vi "Set initial rect size.vi"(8 "error in (no error)":errorcluster, 11 "Cam Session":T1) -> (0 "error out":errorcluster, 2 "Rectangle":T2, 3 "Session Out":T1)   [LabVIEW 2020]
uses:
  <vilib>/vision/driver/NI_Vision_Acquisition_Software.lvlib
  <vilib>/userDefined/High Color/IMAQdx.ctl
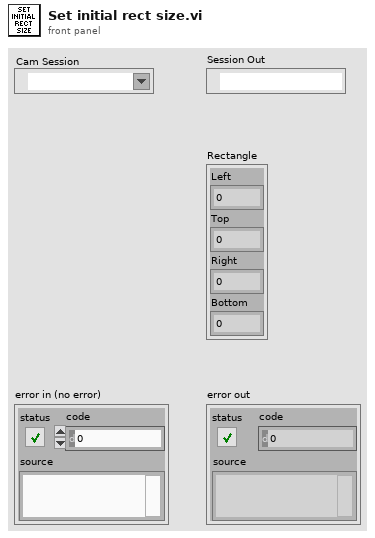
[diagram p1: front panel]
types:
  T1 = typedef "IMAQdx.ctl" = refnum<k21>
  T2 = cluster{"Left":i32, "Top":i32, "Right":i32, "Bottom":i32}
  T3 = typedef "IMAQ Image.ctl" = refnum<image>
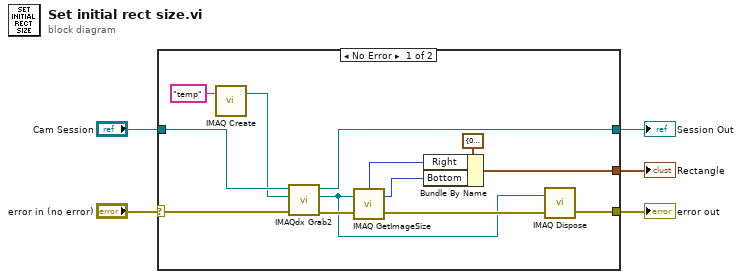
[diagram p0: block diagram]
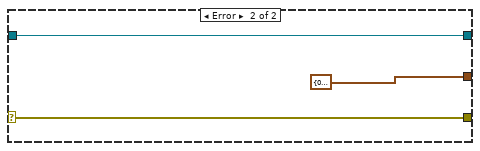
[diagram p2: hidden frame]
diagram:
  n1 = case shown="No Error" "error in (no error)" {
    selector: "error in (no error)" -> [w17 w21]
    tunnel: [w7 w21] -> w4
    tunnel: "Cam Session" -> [w16 w20]
    tunnel: [w14 w20] -> w2
    tunnel: [w9 T2 {"Left"=0, "Top"=0, "Right"=0, "Bottom"=0} ("Rectangle")] -> w1
    frame No Error {
      n2 = call "IMAQ Create"("Image Name"="temp") -> ("New Image"=w15:T3)  [unwired: 4 in, 1 out]
      n3 = call <vilib>:"IMAQdx Grab2.vi"("error in"=w17, "Image In"=w15, "Session In"=w16) -> ("error out"=w13:errorcluster, "Image Out"=w6:T3, "Session Out"=w14:T1)  [unwired: 5 in, 1 out]
      n4 = call "IMAQ GetImageSize"("Image"=w6, "error in (no error)"=w13) -> ("Y Resolution"=w10:i32, "X Resolution"=w11:i32, "error out"=w8:errorcluster)  [unwired: 2 in]
      n5 = Bundle By Name(cluster=T2 {"Left"=0, "Top"=0, "Right"=0, "Bottom"=0} ("Rectangle"), "Right"=w11, "Bottom"=w10) -> (w9:T2)
      n6 = call "IMAQ Dispose"("Image"=w6, "error in (no error)"=w8) -> ("error out"=w7:errorcluster)  [unwired: 4 in]
    }
    frame Error {
    }
  }
  "Rectangle" <- w1
  "error out" <- w4
  "Session Out" <- w2
